vi "TEST_bench_K_times__X_minus_Nx_times_ye__singleAxis.vi"(6 "NS + 1":u8=9, 8 "xk_1_2_mem":fxp<+/-,32,5>[](array[numeric])=[0.0, 0.0, 0.0, 0.0, 0.0, 0.0, 0.0, 0.0, 0.0, 0.0, 0.0, 0.0, 0.0, 0.0, 0.0, 0.0, 0.0, 0.0, 0.0, 0.0, 0.0, 0.0, 0.0, 0.0, 0.0, 0.0, 0.0, 0.0, 0.0, 0.0, 0.0, 0.0, 0.0, 0.0, 0.0, 0.0, 0.0, 0.0, 0.0, 0.0, 0.0, 0.0, 0.0, 0.0, 0.0, 0.0, 0.0, 0.0, 0.0, 0.0], 11 "Nx":fxp<+/-,32,5>[](array[numeric])=[0.0, 0.0, 0.0, 0.0, 0.0, 0.0, 0.0, 0.0, 0.0, 0.0, 0.0, 0.0, 0.0, 0.0, 0.0, 0.0, 0.0, 0.0, 0.0, 0.0, 0.0, 0.0, 0.0, 0.0, 0.0, 0.0, 0.0, 0.0, 0.0, 0.0, 0.0, 0.0, 0.0, 0.0, 0.0, 0.0, 0.0, 0.0, 0.0, 0.0, 0.0, 0.0, 0.0, 0.0, 0.0, 0.0, 0.0, 0.0, 0.0, 0.0]) -> ()   [LabVIEW 2017]
uses:
  fpga_subVIs_ssxy/fixed-point-ss/typeDefs/Kz_vec_scalar.ctl
  fpga_subVIs_ssxy/fixed-point-ss/typeDefs/Kz_bram.ctl
  fpga_subVIs_ssxy/fixed-point-ss/typeDefs/Nx_bram.ctl
  fpga_subVIs_ssxy/fixed-point-ss/typeDefs/x_vec_bram.ctl
  <vilib>/rvi/DataTransferAndStorage/Container/Common/niFpgaContainerExecOnDevCompGetState.vi
  <vilib>/rvi/Emulation/niFpgaEmulationIsFPGAContextNoSignature.vi
  <vilib>/rvi/DataTransferAndStorage/Container/Common/niFpgaContainerGetUniqueNameForEmu.vi
  <vilib>/rvi/Emulation/niFpgaProcessEmulError.vi
  <vilib>/rvi/Emulation/niFpgaSctlEmulationGetInTimedLoop.vi
  <vilib>/rvi/errors/nirviReportUnexpectedCaseInternalError (U32).vi
  <vilib>/rvi/Memory/Memory_Emulation/niFpgaMemoryEmulationCacheClearOnFirstRun.vi
  <vilib>/rvi/Memory/Memory_Emulation/nirvimemoryEmulationManagerCache_MakeExclusive.vi
  <vilib>/rvi/Memory/Memory_Emulation/niFpgaMemoryEmulationValidateCache.vi
  <vilib>/rvi/Memory/Memory_Emulation/nirvimemoryEmulationManagerCache_InsertValue.vi
  <vilib>/Utility/error.llb/Clear Errors.vi
  <vilib>/rvi/Memory/Memory_Emulation/nirvimemoryEmulationManagerCache_ReleaseExclusive.vi
  <vilib>/rvi/Memory/Memory_Emulation/nirvimemoryEmulationManagerCache_GetValue.vi
  <vilib>/rvi/Memory/Memory_Emulation/nirvimemoryEmulationManagerCache_SetValue.vi
  <vilib>/rvi/Emulation/niFpgaSctlEmulationResourceMgr.vi
  <vilib>/rvi/DataTransferAndStorage/Container/XNode/niFpgaContainer.xnode
  <vilib>/rvi/Memory/Memory_Emulation/niFpgaMemoryEmulationRefIn.vi
panel:
  out "uk(expected)":fxp<+/-,32,16>
  in  "K":T1[](array[typedef])=[0.0, 0.0, 0.0, 0.0, 0.0, 0.0, 0.0, 0.0, 0.0, 0.0, 0.0, 0.0, 0.0, 0.0, 0.0, 0.0, 0.0, 0.0, 0.0, 0.0, 0.0, 0.0, 0.0, 0.0, 0.0, 0.0, 0.0, 0.0, 0.0, 0.0, 0.0, 0.0, 0.0, 0.0, 0.0, 0.0, 0.0, 0.0, 0.0, 0.0, 0.0, 0.0, 0.0, 0.0, 0.0, 0.0, 0.0, 0.0, 0.0, 0.0]
  out "x0_expected":fxp<+/-,64,11>[](array[numeric])
  in  "yd_est_x":fxp<+/-,32,5>
  in  "ref(k)_x":fxp<+/-,32,5>
  out "u(k)":fxp<+/-,32,16>
  # "Test that\nxk_1_2 - (r - yd)*Nx"
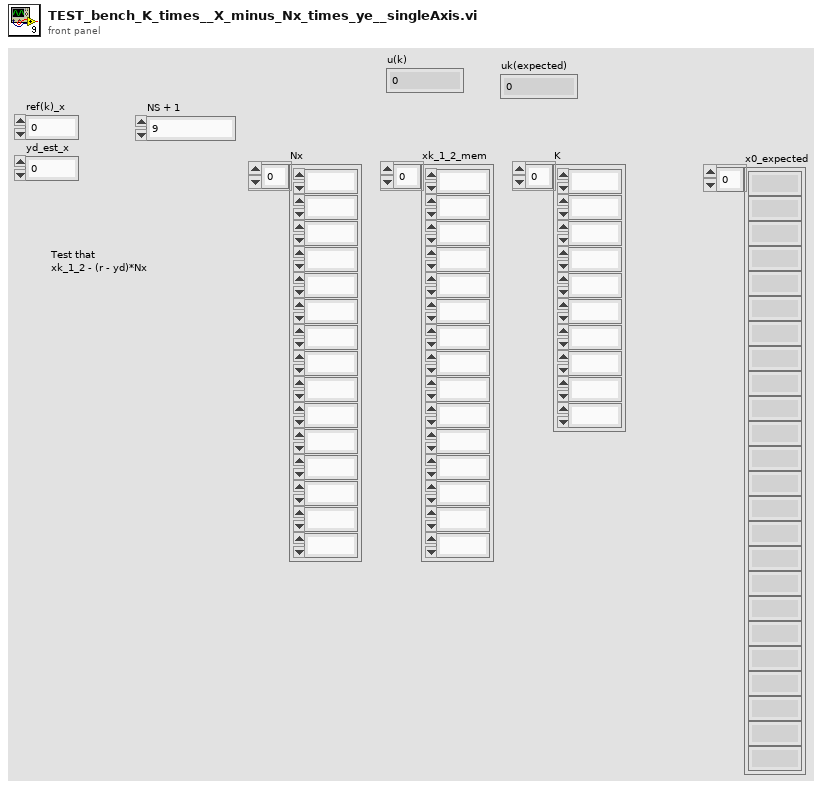
[diagram p1: front panel]
types:
  T1 = typedef "Kz_vec_scalar.ctl" = fxp<+/-,32,10>
  T2 = typedef "Kz_bram.ctl" = refnum<k21>
  T3 = typedef "Nx_bram.ctl" = refnum<k21>
  T4 = typedef "x_vec_bram.ctl" = refnum<k21>
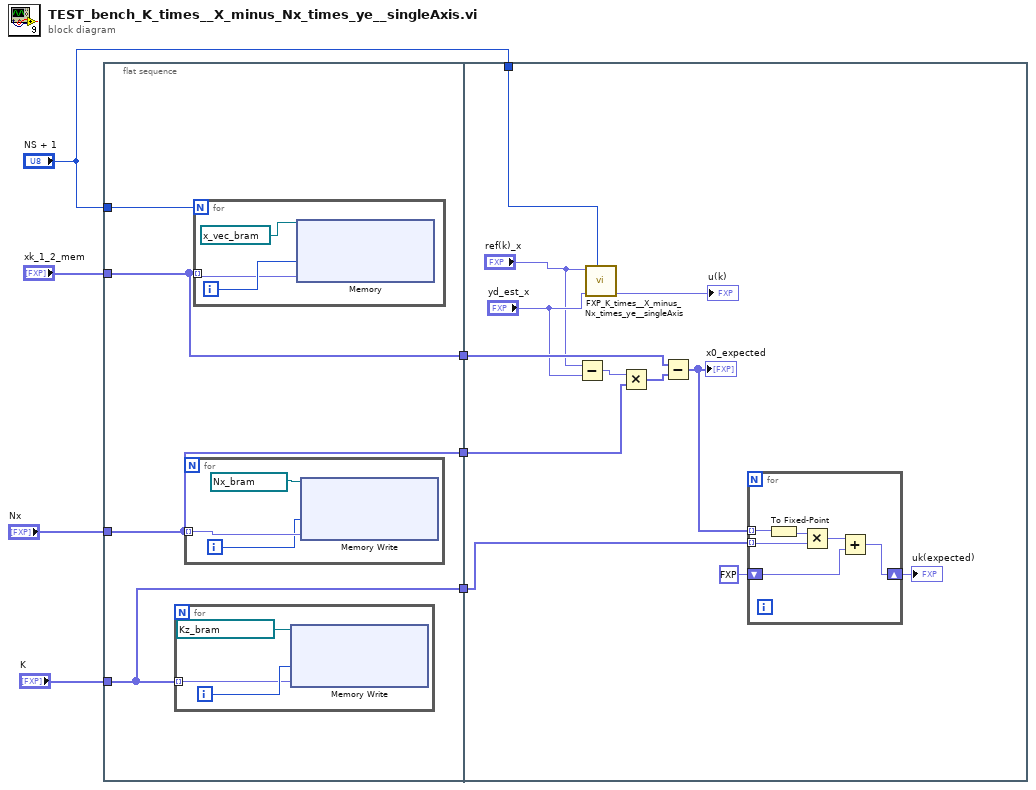
[diagram p0: block diagram]
diagram:
  n1 = flat-sequence {
    tunnel: "NS + 1" -> [w11]
    tunnel: "xk_1_2_mem" -> [w9]
    tunnel: "Nx" -> [w10]
    tunnel: [w10] -> w4
    tunnel: [w9] -> w3
    tunnel: "K" -> [w8]
    tunnel: [w8] -> w1
    tunnel: "NS + 1" -> [w24]
    tunnel: w4 -> [w31]
    tunnel: w3 -> [w29]
    tunnel: w1 -> [w28]
    frame #0 {
      n2 = for {
        tunnel: w8 -> [w12] mode=indexing
        i -> [w13]
        n3 = xnode "Memory Write"("Address"=w13, "Data"=w12, "Memory In"=T2 "K_FXP_row1" ("Memory")) -> ()  [unwired: 1 out]
      }
      n4 = for {
        tunnel: w10 -> [w17] mode=indexing
        i -> [w16]
        n5 = xnode "Memory Write"("Address"=w16, "Data"=w17, "Memory In"=T3 "Nx_col1" ("Nx")) -> ()  [unwired: 1 out]
      }
      n6 = for {
        N: w11 -> [_]
        tunnel: w9 -> [w19] mode=indexing
        i -> [w20]
        n7 = xnode "Memory"("Address"=w20, "Data"=w19, "Memory In"=T4 "xk_1_2" ("Memory")) -> ()  [unwired: 1 out]
      }
    }
    frame #1 {
      n8 = Subtract(x="ref(k)_x", y="yd_est_x") -> (x-y=w32:fxp<+/-,33,6>)
      n9 = call "FXP_K_times__X_minus_Nx_times_ye__singleAxis.vi"("NS"=w24, "yd_est_x"="yd_est_x", "ref(k)_x"="ref(k)_x") -> ("K*xerr"=→"u(k)":fxp<+/-,32,16>)  [unwired: 8 in]
      n10 = Multiply(x=w32, y=w31) -> (x*y=w30:fxp<+/-,64,10>[])
      n11 = Subtract(x=w29, y=w30) -> (x-y=w27:fxp<+/-,32,5>[])
      "x0_expected" <- w27
      n12 = for {
        tunnel: w28 -> [w38] mode=indexing
        tunnel: w27 -> [w34] mode=indexing
        shift-right: [w36] -> w25
        shift-left: fxp<+/-,32,16> 0.0 -> [w37]
        n13 = To Fixed-Point(number=w34) -> (fixed-point=w35:fxp<+/-,32,6>)  [unwired: 1 in]
        n14 = Multiply(x=w35, y=w38) -> (x*y=w33:fxp<+/-,64,16>)
        n15 = Add(x=w33, y=w37) -> (x+y=w36:fxp<+/-,32,16>)
      }
      "uk(expected)" <- w25
    }
  }
